vi "Check Password.vi"(8 "error in (no error)":errorcluster, 11 "TCP Network Connection in":refnum<k5>) -> (0 "error out":errorcluster, 2 "Authorized Level":enum16{"Read Only", "Operator", "Admin"}(ring), 3 "connection ID out":refnum<k5>)   [LabVIEW 2020]
doc: "Author: Scott Hannahs <sth@magnet.fsu.edu>\nCopyright 2018 Florida State University, All rights reserved."
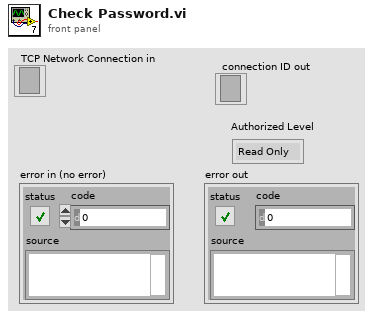
[diagram p1: front panel]
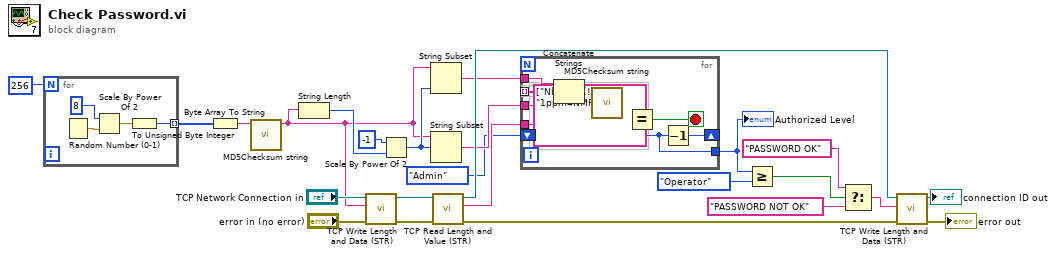
[diagram p0: block diagram]
diagram:
  n1 = for {
    N: 256 -> [_]
    tunnel: [w27] -> w25 mode=indexing
    n2 = Random Number (0-1)() -> (number: 0 to 1=w30:dbl)
    n3 = Scale By Power Of 2(n=i16 8, x=w30) -> (x*2^n=w28:dbl)
    n4 = To Unsigned Byte Integer(number=w28) -> (unsigned 8bit integer=w27:u8)
  }
  n5 = Byte Array To String(unsigned byte array=w25) -> (string=w24:string)
  n6 = call <vilib>:"MD5Checksum string.vi"("Message String"=w24) -> ("MD5 message-digest"=w10:string)  [unwired: 10 in]
  n7 = String Length(string=w10) -> (length=w13:i32)
  n8 = call "TCP Write Length and Data (STR).vi"("Error In"="error in (no error)", "Data"=w10, "connection ID"="TCP Network Connection in") -> ("Error Out"=w21:errorcluster, "connection ID out"=w20:refnum<k5>)  [unwired: 7 in]
  n9 = Scale By Power Of 2(n=i16 -1, x=w13) -> (x*2^n=w11:i32)
  n10 = String Subset(string=w10, length (rest)=w11) -> (substring=w8:string)  [unwired: 1 in]
  n11 = String Subset(string=w10, offset (0)=w11) -> (substring=w7:string)  [unwired: 1 in]
  n12 = call "TCP Read Length and Value (STR).vi"("error in (no error)"=w21, "TCP Network Connection in"=w20) -> ("error out"=w19:errorcluster, "Output"=w6:string, "TCP Network Connection out"=w17:refnum<k5>)  [unwired: 7 in]
  n13 = for {
    tunnel: string[] ["Nb3$n<(!((", "1ppm4NMR!", " "] -> [w39] mode=indexing
    tunnel: w8 -> [w38]
    tunnel: w7 -> [w37]
    tunnel: w6 -> [w34]
    shift-right: [w31] -> _
    shift-left: enum16{"Read Only", "Operator", "Admin"}."Admin" ("Authorized Level") -> [w32]
    tunnel: [w32] -> w4
    stop <- w33 stop-if-true
    n14 = Concatenate Strings(w38, w39, w37) -> (w36:string)
    n15 = call <vilib>:"MD5Checksum string.vi"("Message String"=w36) -> ("MD5 message-digest"=w35:string)  [unwired: 10 in]
    n16 = Equal?(x=w35, y=w34) -> (x = y?=w33:bool)
    n17 = Decrement(x=w32) -> (x-1=w31:enum16{"Read Only", "Operator", "Admin"})
  }
  "Authorized Level" <- w4
  n18 = Greater Or Equal?(x=w4, y=enum16{"Read Only", "Operator", "Admin"}."Operator") -> (x >= y?=w2:bool)
  n19 = Select(t="PASSWORD OK" ("Data"), s=w2, f="PASSWORD NOT OK") -> (s? t:f=w16:string)
  n20 = call "TCP Write Length and Data (STR).vi"("Error In"=w19, "Data"=w16, "connection ID"=w17) -> ("Error Out"=→"error out":errorcluster, "connection ID out"=→"connection ID out":refnum<k5>)  [unwired: 7 in]
